vi "Create SQL Update Top (1) Set Clause.vi"(6 "Data Types":enum16{"String", "Number", "Date-Time"}[](array[ring])=[enum."String", enum."String", enum."String", enum."String", enum."String", enum."String", enum."Number", enum."Number", enum."Date-Time", enum."String", enum."Number", enum."Number", enum."String", enum."Number", enum."Number", enum."Date-Time", enum."Date-Time", enum."String"], 8 "Where Clause":string, 9 "New Data (Strings)":string[](array[string]), 10 "Column Headers":string[](array[string]), 11 "Table to Update":string) -> (3 "SET Statement":string)   [LabVIEW 2010]
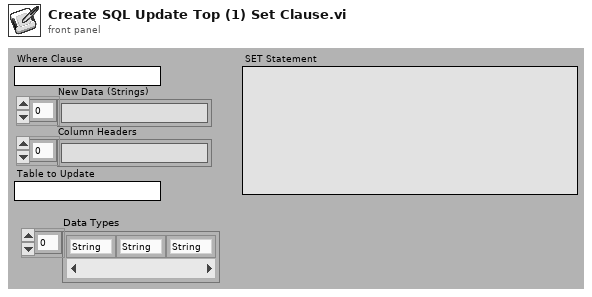
[diagram p1: front panel]
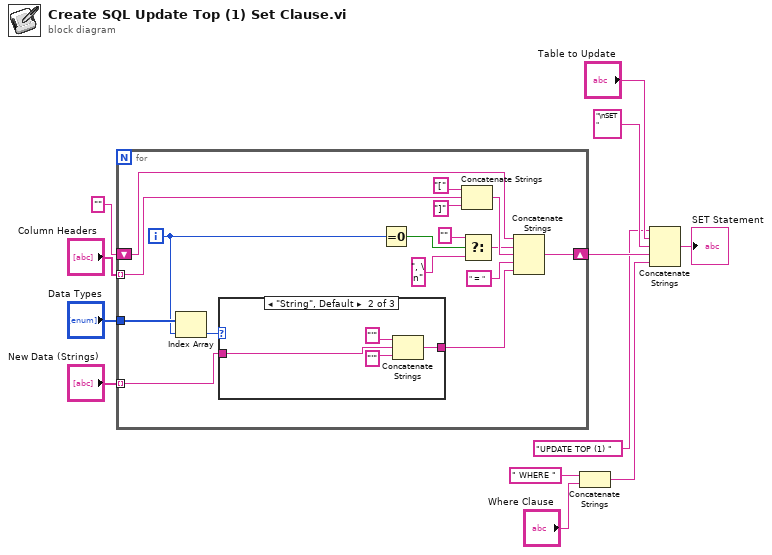
[diagram p0: block diagram]
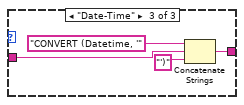
[diagram p3: hidden frame]
diagram:
  n1 = for {
    tunnel: "New Data (Strings)" -> [w28] mode=indexing
    shift-right: [w25] -> w10
    shift-left: "" -> [w17]
    tunnel: "Column Headers" -> [w24] mode=indexing
    tunnel: "Data Types" -> [w15]
    i -> [w14]
    n2 = Index Array(array=w15, index=w14) -> (element=w13:enum16{"String", "Number", "Date-Time"})
    n3 = case shown="\"String\", Default" w13 {
      tunnel: w28 -> [w29 w31 w35]
      tunnel: [w29 w30 w34] -> w27
      frame "Number" {
      }
      frame "String", Default {
        n4 = Concatenate Strings("'" ("string"), w31, "'" ("string")) -> (w30:string)
      }
      frame "Date-Time" {
        n5 = Concatenate Strings("CONVERT (Datetime, '" ("string"), w35, "')" ("string")) -> (w34:string)
      }
    }
    n6 = Equal To 0?(x=w14) -> (x = 0?=w20:bool)
    n7 = Concatenate Strings("[" ("string"), w24, "]" ("string")) -> (w21:string)
    n8 = Select(t="", s=w20, f=", \n" ("string")) -> (s? t:f=w16:string)
    n9 = Concatenate Strings(w17, w16, w21, " = " ("string"), w27) -> (w25:string)
  }
  n10 = Concatenate Strings(" WHERE " ("string"), "Where Clause") -> (w12:string)
  n11 = Concatenate Strings("UPDATE TOP (1) " ("string"), "Table to Update", "\nSET " ("string"), w10, w12) -> (→"SET Statement":string)
